vi "Write Target Destination VI.vi"(8 "error in (no error)":errorcluster, 10 "Target Destination VI":path, 11 "RIO Target Configuration in":refnum<class "RIO Target Configuration.lvclass">) -> (0 "error out":errorcluster, 3 "RIO Target Configuration out":refnum<class "RIO Target Configuration.lvclass">)   [LabVIEW 2014, in "RIO Target Configuration.lvclass"]
uses:
  RIO Target Configuration.lvclass
  RIO Target Configuration.lvclass/RIO Target Configuration.ctl
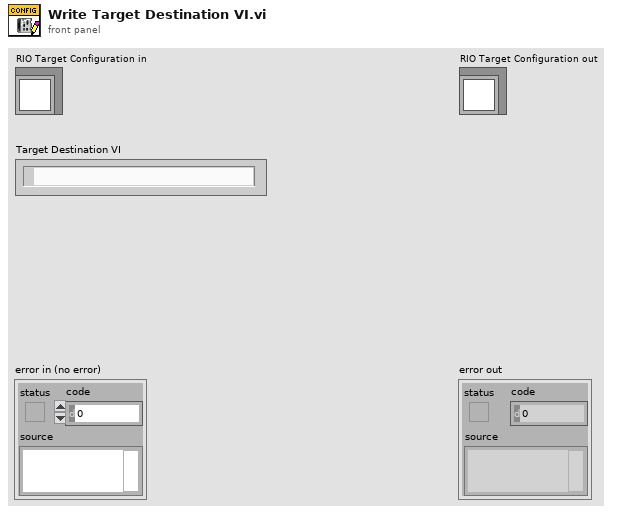
[diagram p1: front panel]
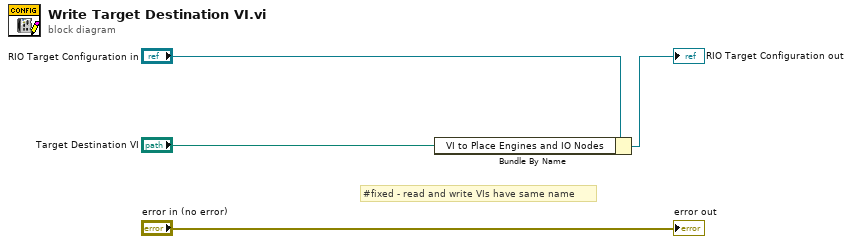
[diagram p0: block diagram]
diagram:
  # "#fixed - read and write VIs have same name"
  n1 = Bundle By Name(cluster="RIO Target Configuration in", "VI to Place Engines and IO Nodes"="Target Destination VI") -> (→"RIO Target Configuration out":refnum<class "RIO Target Configuration.lvclass">)
  "error out" <- "error in (no error)"
